vi "ServoTempRead.vi"(10 "ID":u8=1) -> (2 "Command":string)   [LabVIEW 2013]
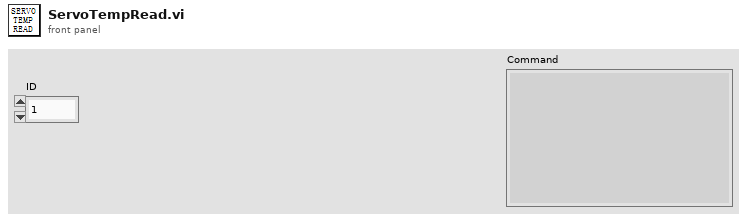
[diagram p1: front panel]
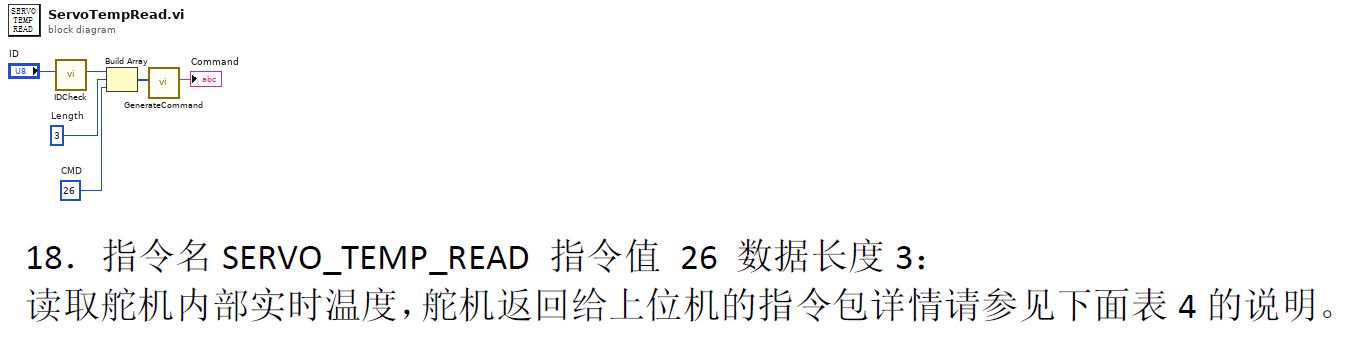
[diagram p0: block diagram]
diagram:
  w3 = u8 26  # CMD
  w4 = u8 3  # Length
  n1 = call "IDCheck.vi"("IDIn"="ID") -> ("IDOut"=w5:u8)  [unwired: 10 in]
  n2 = Build Array(w5, w4, w3) -> (w2:u8[])
  n3 = call "GenerateCommand.vi"("DataIn"=w2) -> ("Command"=→"Command":string)  [unwired: 10 in]
